vi "Write MonoCommunicator.vi"(8 "error in (no error)":errorcluster, 10 "MonoCommunicator.lvclass":refnum<class "MonoCommunicator.lvclass">, 11 "Monochromator in":refnum<class "Monochromator.lvclass">) -> (0 "error out":errorcluster, 3 "Monochromator out":refnum<class "Monochromator.lvclass">)   [LabVIEW 2016, in "Monochromator.lvclass"]
uses:
  Monochromator.lvclass
  MonoCommunicator/MonoCommunicator.lvclass
  Monochromator.lvclass/Monochromator.ctl
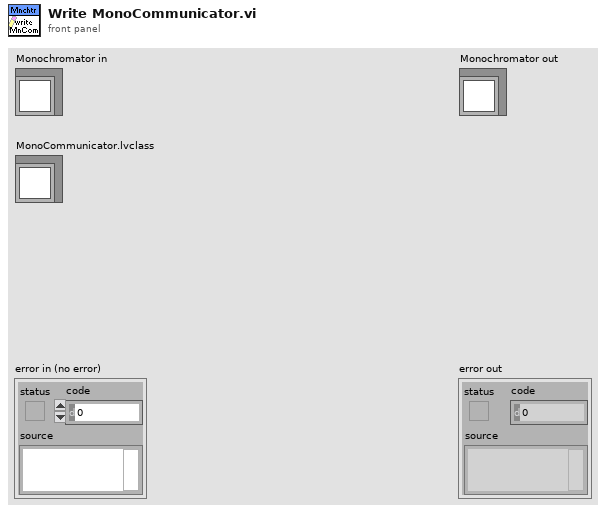
[diagram p1: front panel]
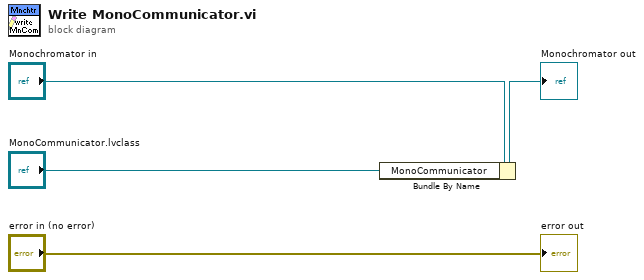
[diagram p0: block diagram]
diagram:
  n1 = Bundle By Name(cluster="Monochromator in", "MonoCommunicator"="MonoCommunicator.lvclass") -> (→"Monochromator out":refnum<class "Monochromator.lvclass">)
  "error out" <- "error in (no error)"
